vi "SavedSignal.vi"(11 "File selected":T2) -> (1 "Settings out":T1={"Name of test"="", "Date"=timestamp(0 s since 1904-01-01), "Location"="", "Template"="", "Soundcard"="", "resolution"=32, "Sampling rate"=48000, "Ch1 Gain "=0.0, "Ch2 Gain"=0.0, "Sample time (s)"=0.3, "Pre-trigger (s)"=0.01, "Hammer Threshold"=0.01, "Positions"=12, "Taps/Position"=5, "Set Names"="", "Freq resolution"=1.0, "Hammer cutoff"=1.0, "Mic cutoff"=1.0, "Double bounce "=0.0, "Hammer Cal"=1.0, "dB Offset"=0.0, "Accel Cal"=10.0, "Vibrometer Cal"=0.0, "Mic Cal"=1.0, "Output"=2, "Voltage Cal"=1.0, "Vibrometer Port"="ASRL27::INSTR", "Range"=10, "High Pass"=2, "Bandwidth"=25, "X Range"=[], "Y Range"=[], "dB Spread"=40.0, "Trigger"=0, "Ch_1"=1, "Ch_2"=2, "flip?"=FALSE, "60Hz"=FALSE, "Time offset"=0.0, "Piezo Cal"=1.0, "Default Notes"=""} {"Ch_2" min=1 step=1; "Ch_1" min=1 max=100 step=1; "Trigger" items=["Hammer (force)", "Self-tap", "Spacebar"]; "Bandwidth" items=["1 kHz"=1, "5 kHz"=5, "10 kHz"=10, "25 kHz"=25, "50 kHz"=50, "100 kHz"=100]; "High Pass" items=["Off", "13 Hz", "104 Hz"]; "Range" items=["10 mm/s"=1, "20 mm/s"=2, "50 mm/s"=5, "100 mm/s"=10, "200 mm/s"=20, "500 mm/s"=50, "1 m/s"=100, "2 m/s"=200]; "Output" items=["Accelerometer", "Speed (from acceleration)", "Microphone", "Vibrometer", "Piezo"]; "Voltage Cal" format="%#_13g"; "Ch2 Gain" format="%#_13g"; "Ch1 Gain" format="%#_13g"; "Double bounce" min=0.0; "Mic cutoff" min=0.0 format="%#_4g"; "Hammer cutoff" min=0.0 format="%#_4g"; "Freq resolution" min=0.0; "Pre-trigger (s)" format="%#_13g"; "Date" format="%<%H:%M\n%d/%m/%y>T"; "resolution" items=["16 bit"=16, "24 bit"=24, "32 bit"=32]; "Sampling rate" items=["22050 samp/s"=22050, "44100 samp/s"=44100, "48000 samp/s"=48000]}, 3 "update?":bool)   [LabVIEW 2022 SP3]
uses:
  ViolinSubs/PreferencesControl.ctl
  ViolinSubs/Curtin1_Label.ctl
  ViolinSubs/Mic/Mic_Global.vi
panel:
  out "Complex FRF":cluster{dbl, "df":dbl, cdb[]}
  out "starting settings":T1={"Name of test"="", "Date"=timestamp(0 s since 1904-01-01), "Location"="", "Template"="", "Soundcard"="", "resolution"=0, "Sampling rate"=0, "Ch1 Gain "=0.0, "Ch2 Gain"=0.0, "Sample time (s)"=0.0, "Pre-trigger (s)"=0.0, "Hammer Threshold"=0.0, "Positions"=0, "Taps/Position"=0, "Set Names"="", "Freq resolution"=0.0, "Hammer cutoff"=0.0, "Mic cutoff"=0.0, "Double bounce "=0.0, "Hammer Cal"=0.0, "dB Offset"=0.0, "Accel Cal"=0.0, "Vibrometer Cal"=0.0, "Mic Cal"=0.0, "Output"=0, "Voltage Cal"=0.0, "Vibrometer Port"="", "Range"=0, "High Pass"=0, "Bandwidth"=0, "X Range"=[], "Y Range"=[], "dB Spread"=0.0, "Trigger"=0, "Ch_1"=0, "Ch_2"=0, "flip?"=FALSE, "60Hz"=FALSE, "Time offset"=0.0, "Piezo Cal"=1.0, "Default Notes"=""} {"Ch_2" min=1 step=1; "Ch_1" min=1 max=100 step=1; "Trigger" items=["Hammer (force)", "Self-tap", "Spacebar"]; "Bandwidth" items=["1 kHz"=1, "5 kHz"=5, "10 kHz"=10, "25 kHz"=25, "50 kHz"=50, "100 kHz"=100]; "High Pass" items=["Off", "13 Hz", "104 Hz"]; "Range" items=["10 mm/s"=1, "20 mm/s"=2, "50 mm/s"=5, "100 mm/s"=10, "200 mm/s"=20, "500 mm/s"=50, "1 m/s"=100, "2 m/s"=200]; "Output" items=["Accelerometer", "Speed (from acceleration)", "Microphone", "Vibrometer", "Piezo"]; "Voltage Cal" format="%#_13g"; "Ch2 Gain" format="%#_13g"; "Ch1 Gain" format="%#_13g"; "Double bounce" min=0.0; "Mic cutoff" min=0.0 format="%#_4g"; "Hammer cutoff" min=0.0 format="%#_4g"; "Freq resolution" min=0.0; "Pre-trigger (s)" format="%#_13g"; "Date" format="%<%H:%M\n%d/%m/%y>T"; "resolution" items=["16 bit"=16, "24 bit"=24, "32 bit"=32]; "Sampling rate" items=["22050 samp/s"=22050, "44100 samp/s"=44100, "48000 samp/s"=48000]}
  out "path to settings file":path
  in  "Save as a Template":bool
  in  "Offset (msec)":dbl(slide) scale=0.0..10.0
  out "data":waveform(dbl)[](array[waveform])
  in  "Tab Control":enum32{"Raw", "Raw Calibrated", "Zoomed in"}(tab)
  out "Hammer":waveform(dbl)[](graph)
  out "Microphone":waveform(dbl)[](graph)
  out "Cal Hammer":waveform(dbl)[](graph)
  out "cal Mic":waveform(dbl)[](graph)
  out "Trig Mic":waveform(dbl)[](graph)
  out "Trig Hammer":waveform(dbl)[](graph)
  out "Average FRF":cluster{dbl, "df":dbl, dbl[]}(graph)
  out "Real/Imag":cluster{dbl, "df":dbl, dbl[]}[](graph)
  in  "Settings":T1={"Name of test"="", "Date"=timestamp(0 s since 1904-01-01), "Location"="", "Template"="", "Soundcard"="", "resolution"=32, "Sampling rate"=48000, "Ch1 Gain "=0.0, "Ch2 Gain"=0.0, "Sample time (s)"=0.3, "Pre-trigger (s)"=0.01, "Hammer Threshold"=0.01, "Positions"=12, "Taps/Position"=5, "Set Names"="", "Freq resolution"=1.0, "Hammer cutoff"=1.0, "Mic cutoff"=1.0, "Double bounce "=0.0, "Hammer Cal"=1.0, "dB Offset"=0.0, "Accel Cal"=10.0, "Vibrometer Cal"=0.0, "Mic Cal"=1.0, "Output"=2, "Voltage Cal"=1.0, "Vibrometer Port"="ASRL27::INSTR", "Range"=10, "High Pass"=2, "Bandwidth"=25, "X Range"=[], "Y Range"=[], "dB Spread"=40.0, "Trigger"=0, "Ch_1"=1, "Ch_2"=2, "flip?"=FALSE, "60Hz"=FALSE, "Time offset"=0.0, "Piezo Cal"=1.0, "Default Notes"=""} {"Ch_2" min=1 step=1; "Ch_1" min=1 max=100 step=1; "Trigger" items=["Hammer (force)", "Self-tap", "Spacebar"]; "Bandwidth" items=["1 kHz"=1, "5 kHz"=5, "10 kHz"=10, "25 kHz"=25, "50 kHz"=50, "100 kHz"=100]; "High Pass" items=["Off", "13 Hz", "104 Hz"]; "Range" items=["10 mm/s"=1, "20 mm/s"=2, "50 mm/s"=5, "100 mm/s"=10, "200 mm/s"=20, "500 mm/s"=50, "1 m/s"=100, "2 m/s"=200]; "Output" items=["Accelerometer", "Speed (from acceleration)", "Microphone", "Vibrometer", "Piezo"]; "Voltage Cal" format="%#_13g"; "Ch2 Gain" format="%#_13g"; "Ch1 Gain" format="%#_13g"; "Double bounce" min=0.0; "Mic cutoff" min=0.0 format="%#_4g"; "Hammer cutoff" min=0.0 format="%#_4g"; "Freq resolution" min=0.0; "Pre-trigger (s)" format="%#_13g"; "Date" format="%<%H:%M\n%d/%m/%y>T"; "resolution" items=["16 bit"=16, "24 bit"=24, "32 bit"=32]; "Sampling rate" items=["22050 samp/s"=22050, "44100 samp/s"=44100, "48000 samp/s"=48000]}
  # "Hz"
  # "dB"
  # "dB"
  # "sec"
  # "sec"
  # "mV/Pa"
  # "mV/m/s2"
  # "mV/mm/s"
  # "V/N"
  # "sec"
  # "sec"
  # "mV/N"
  # "a.u."
  # "a.u."
  # "sec"
  # "Hz"
  # "dB"
  # "dB"
  # "sec"
  # "sec"
  # "mV/Pa"
  # "mV/m/s2"
  # "mV/mm/s"
  # "V/N"
  # "sec"
  # "sec"
  # "mV/N"
  # "a.u."
  # "a.u."
  # "sec"
  # "Raw values from the Soundcard"
  # "Calibrated Values"
  # "Hz"
  # "dB"
  # "dB"
  # "sec"
  # "sec"
  # "mV/Pa"
  # "mV/m/s2"
  # "mV/mm/s"
  # "V/N"
  # "sec"
  # "sec"
  # "mV/N"
  # "a.u."
  # "a.u."
  # "sec"
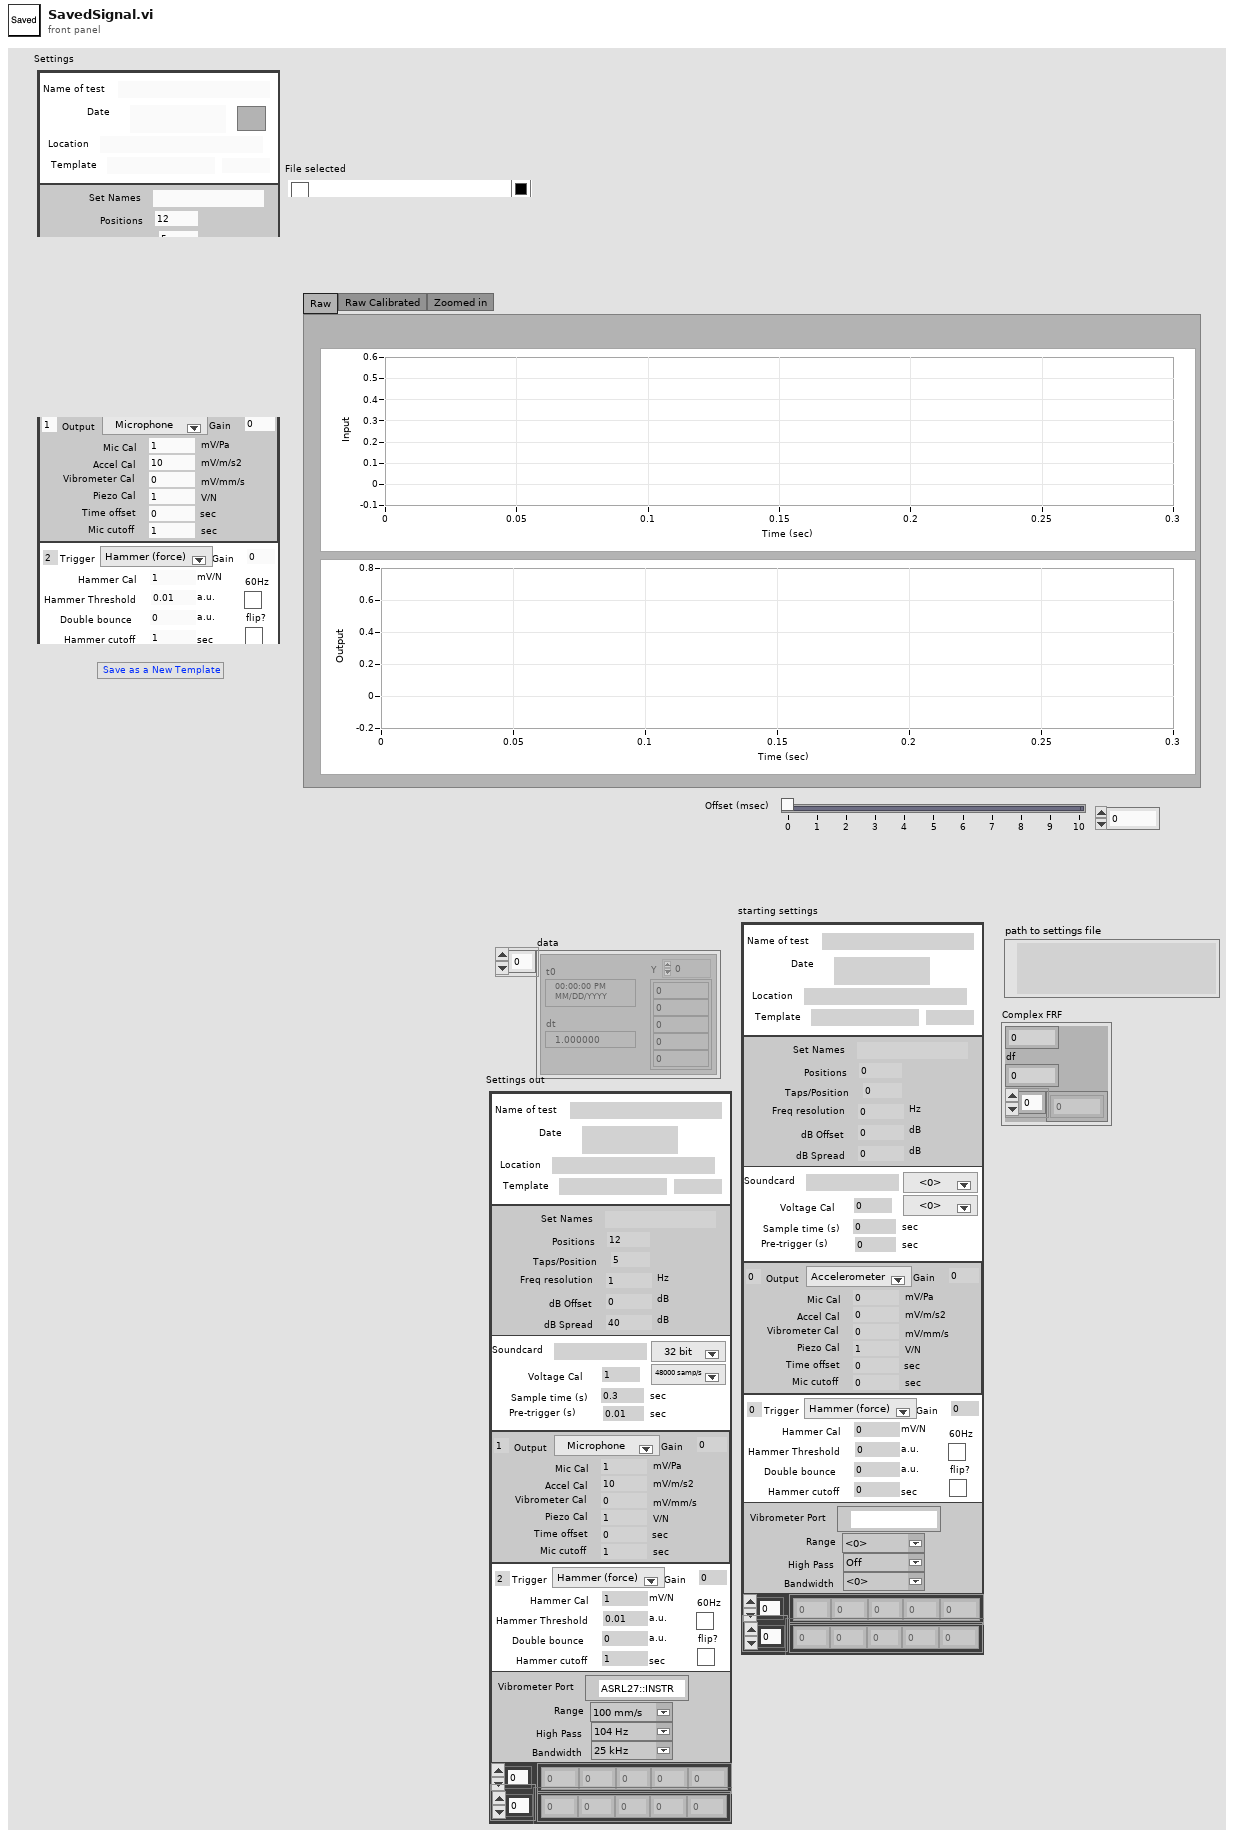
[diagram p1: front panel]
types:
  T1 = typedef "PreferencesControl.ctl" = cluster{"Name of test":string, "Date":timestamp, "Location":string, "Template":string, "Soundcard":string, "resolution":u16, "Sampling rate":u16, "Ch1 Gain ":dbl, "Ch2 Gain":dbl, "Sample time (s)":dbl, "Pre-trigger (s)":dbl, "Hammer Threshold":dbl, "Positions":i16, "Taps/Position":i16, "Set Names":string, "Freq resolution":dbl, "Hammer cutoff":dbl, "Mic cutoff":dbl, "Double bounce ":dbl, "Hammer Cal":dbl, "dB Offset":dbl, "Accel Cal":dbl, "Vibrometer Cal":dbl, "Mic Cal":dbl, "Output":u16, "Voltage Cal":dbl, "Vibrometer Port":refnum<visa-resource-name>, "Range":u16, "High Pass":u16, "Bandwidth":u16, "X Range":cluster{"Minimum":dbl, "Maximum":dbl, "Increment":dbl, "Minor Increment":dbl, "Start":dbl}[], "Y Range":cluster{"Minimum":dbl, "Maximum":dbl, "Increment":dbl, "Minor Increment":dbl, "Start":dbl}[], "dB Spread":dbl, "Trigger":u16, "Ch_1":u8, "Ch_2":u8, "flip?":bool, "60Hz":bool, "Time offset":dbl, "Piezo Cal":dbl, "Default Notes":string}
  T2 = typedef "Curtin1_Label.ctl" = cluster{"Show?":bool, "Name":string, "Color":u32, "Path":path, "Show Notes":bool}
  T3 = enum32{"Invalid", "Default", "Floating", "Floating/Auto-Hide", "Modal"}
  T4 = enum8{"Enabled", "Disabled", "Disabled and Grayed Out"}
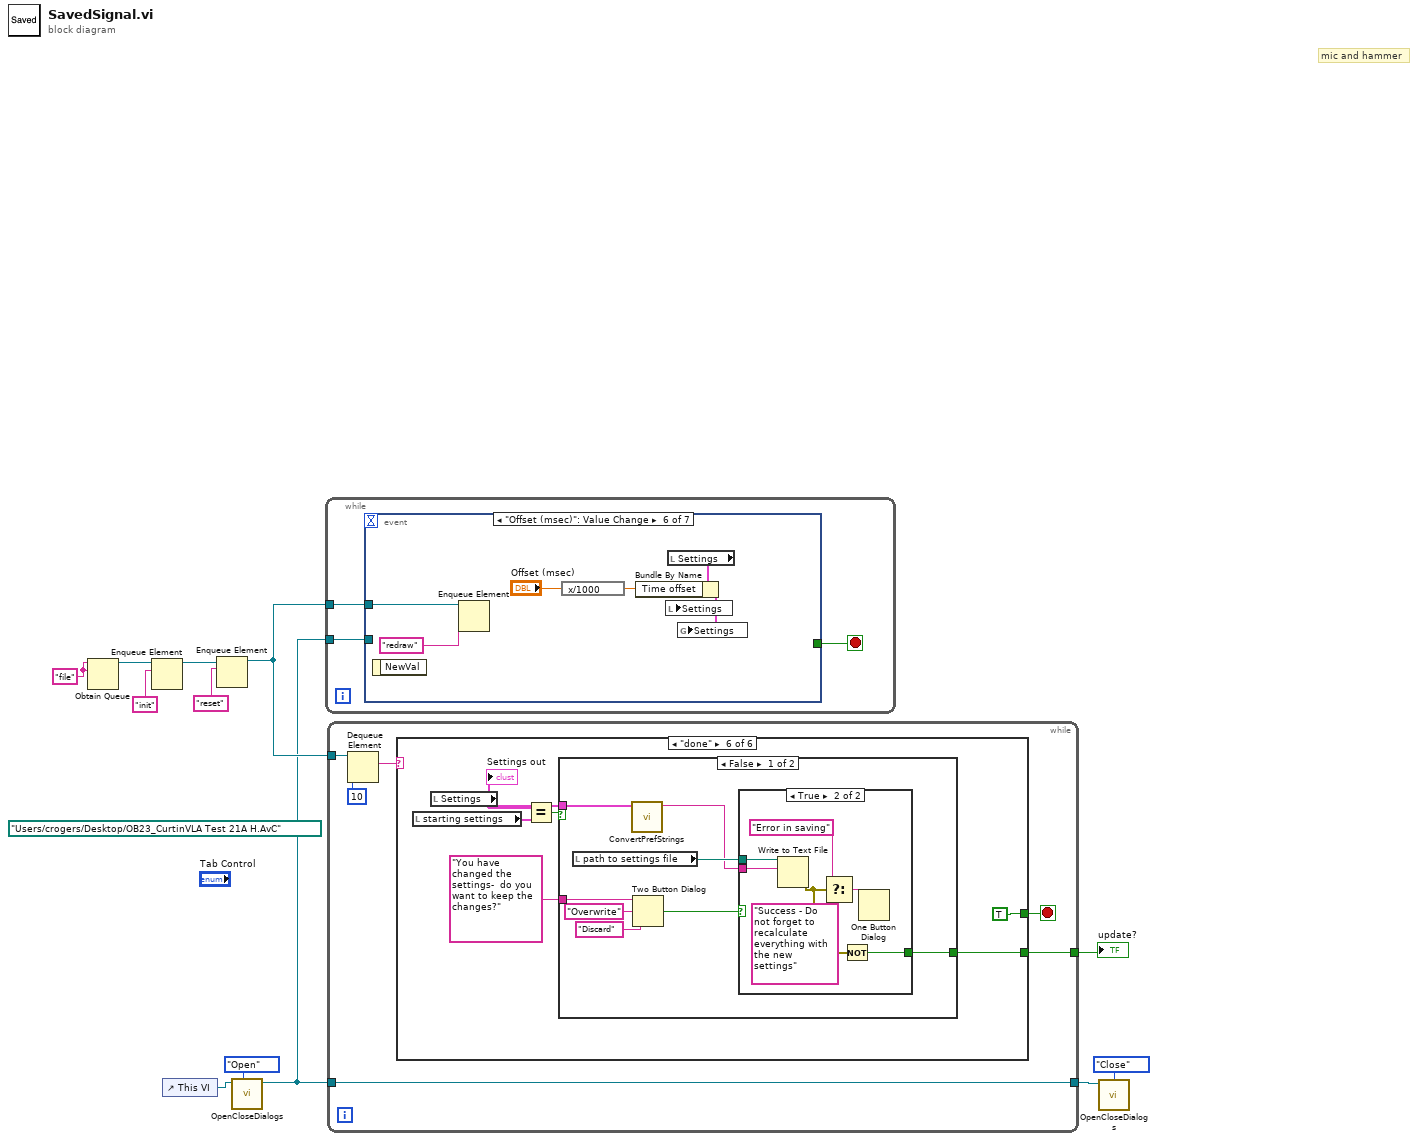
[diagram p0: block diagram]
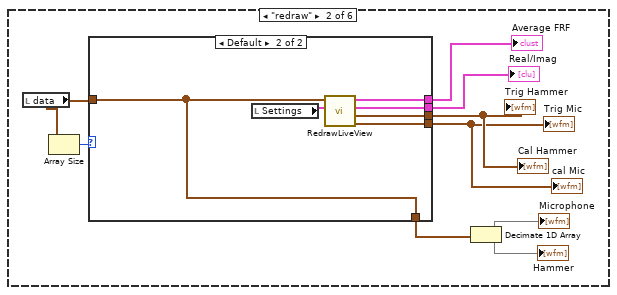
[diagram p3: hidden frame]
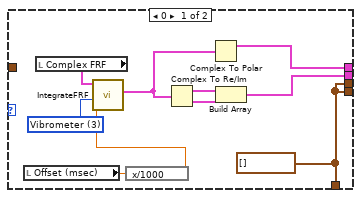
[diagram p4: hidden frame]
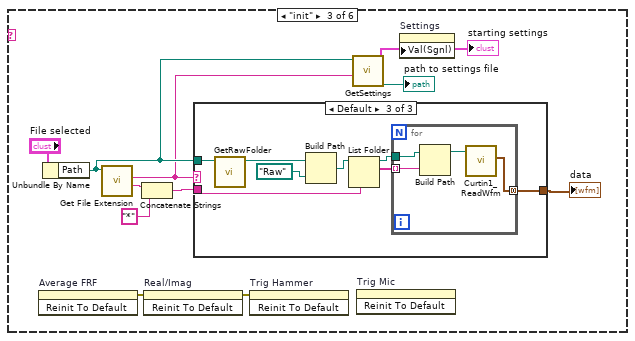
[diagram p5: hidden frame]
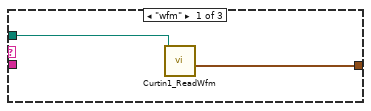
[diagram p6: hidden frame]
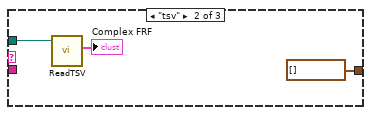
[diagram p7: hidden frame]
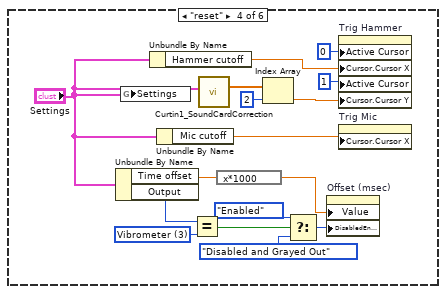
[diagram p8: hidden frame]
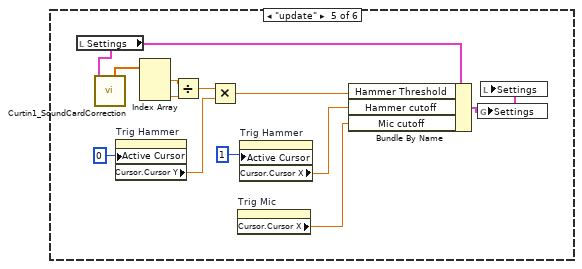
[diagram p9: hidden frame]
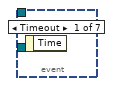
[diagram p12: hidden frame]
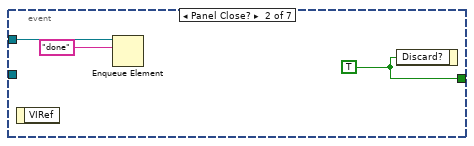
[diagram p13: hidden frame]
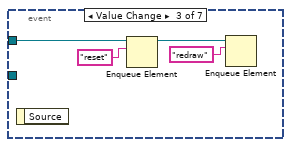
[diagram p14: hidden frame]
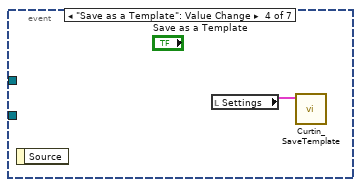
[diagram p15: hidden frame]
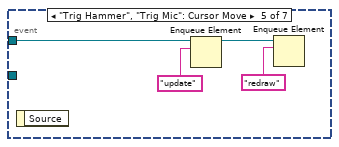
[diagram p16: hidden frame]
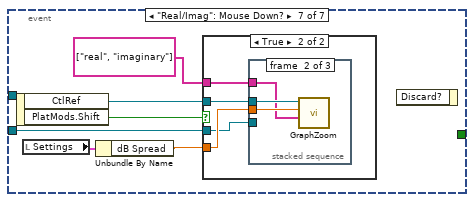
[diagram p17: hidden frame]
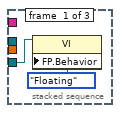
[diagram p19: hidden frame]
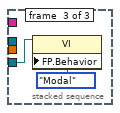
[diagram p20: hidden frame]
diagram:
  (unwired) path "/Users/crogers/Desktop/OB23_CurtinVLA Test 21A H.AvC" ("Path")
  w6 = "file" ("name (unnamed)")
  # "mic and hammer"
  n1 = Obtain Queue(name (unnamed)=w6, element data type=w6) -> (queue out=w5:refnum<queue>)  [unwired: 3 in, 2 out]
  n2 = Enqueue Element(queue=w5, element="init") -> (queue out=w8:refnum<queue>)  [unwired: 2 in, 2 out]
  n3 = control-ref of="This VI"() -> (w3:refnum<vi>)
  n4 = Enqueue Element(queue=w8, element="reset") -> (queue out=w7:refnum<queue>)  [unwired: 2 in, 2 out]
  n5 = call "OpenCloseDialogs.vi"("Task"=enum16{"Open", "Close"}."Open", "VI in"=w3) -> ("VI out"=w2:refnum<vi>)  [unwired: 8 in, 1 out]
  n6 = while {
    tunnel: w7 -> [w15]
    tunnel: w2 -> [w13]
    stop <- w14 stop-if-true
    n7 = event shown="[5] \"Offset (msec)\": Value Change" {
      selector: _ -> [_ _ _ _ _ _ _]
      dyn-events: _ -> [_ _ _ _ _ _ _]
      timeout: _ -> [_ _ _ _ _ _ _]
      tunnel: [_ w18 _ _ _ _ _] -> w14
      tunnel: w15 -> [_ w17 w22 _ w26 w28 _]
      tunnel: w13 -> [_ _ _ _ _ _ w35]
      event Timeout {
        n8 = event-data() -> ()  [unwired: 1 in, 1 out]
      }
      event Panel Close? {
        w18 = TRUE ("Discard?")
        n9 = event-data() -> ()  [unwired: 1 in, 1 out]
        n10 = Enqueue Element(queue=w17, element="done") -> ()  [unwired: 2 in, 3 out]
        n11 = event-data("Discard?"=w18) -> ()  [unwired: 1 in, 1 out]
      }
      event Value Change {
        n12 = event-data() -> ()  [unwired: 1 in, 1 out]
        n13 = Enqueue Element(queue=w22, element="reset") -> (queue out=w20:refnum<queue>)  [unwired: 2 in, 2 out]
        n14 = Enqueue Element(queue=w20, element="redraw") -> ()  [unwired: 2 in, 3 out]
      }
      event "Save as a Template": Value Change {
        n15 = event-data() -> ()  [unwired: 1 in, 1 out]
        n16 = local read "Settings"() -> (w23:T1)
        n17 = call "Curtin_SaveTemplate.vi"("Settings in"=w23) -> ()  [unwired: 8 in, 3 out]
      }
      event "Trig Hammer", "Trig Mic": Cursor Move {
        n18 = event-data() -> ()  [unwired: 1 in, 1 out]
        n19 = Enqueue Element(queue=w26, element="update") -> (queue out=w24:refnum<queue>)  [unwired: 2 in, 2 out]
        n20 = Enqueue Element(queue=w24, element="redraw") -> ()  [unwired: 2 in, 3 out]
      }
      event "Offset (msec)": Value Change {
        n21 = event-data() -> ()  [unwired: 1 in, 1 out]
        n22 = Enqueue Element(queue=w28, element="redraw") -> ()  [unwired: 2 in, 3 out]
        n23 = expression code="x/1000"("Offset (msec)") -> (w30:dbl)
        n24 = local read "Settings"() -> (w33:T1)
        n25 = Bundle By Name(cluster=w33, "Time offset"=w30) -> (w32:T1)
        n26 = local write "Settings"(w32) -> ()
        n27 = global write "Mic_Global.vi" "Settings"(w32) -> ()
      }
      event "Real/Imag": Mouse Down? {
        n28 = event-data() -> ("CtlRef"=w38:refnum<vi>, "PlatMods.Shift"=w39:bool)  [unwired: 1 in]
        n29 = local read "Settings"() -> (w37:T1)
        n30 = Unbundle By Name(w37) -> ("dB Spread"=w36:dbl)
        n31 = case shown="True" w39 {
          tunnel: w38 -> [_ w43]
          tunnel: w36 -> [_ w42]
          tunnel: w35 -> [_ w41]
          tunnel: string[] ["real", "imaginary"] -> [_ w40]
          frame False {
          }
          frame True {
            n32 = stacked-sequence {
              tunnel: w43 -> [_ w48 _]
              tunnel: w42 -> [_ w47 _]
              tunnel: w41 -> [w44 _ w49]
              tunnel: w40 -> [_ w46 _]
              frame #0 {
                n33 = property class="VI"(reference=w44, "FP.Behavior"=T3."Floating" ("Front Panel Window:Behavior")) -> ()  [unwired: 1 in, 2 out]
              }
              frame #1 {
                n34 = call "GraphZoom.vi"("Names"=w46, "dB Range"=w47, "Graph"=w48) -> ()  [unwired: 9 in]
              }
              frame #2 {
                n35 = property class="VI"(reference=w49, "FP.Behavior"=T3."Modal" ("Front Panel Window:Behavior")) -> ()  [unwired: 1 in, 2 out]
              }
            }
          }
        }
        n36 = event-data() -> ()  [unwired: 2 in, 1 out]
      }
    }
  }
  n37 = while {
    tunnel: w7 -> [w56]
    tunnel: [w52] -> w10
    tunnel: w2 -> [w52]
    tunnel: [w51] -> w1
    stop <- w53 stop-if-true
    n38 = Dequeue Element(queue=w56, timeout in ms (-1)=10) -> (element=w55:string)  [unwired: 1 in, 3 out]
    n39 = case shown="\"done\"" w55 {
      tunnel: [_ _ _ _ _ TRUE ("Discard?")] -> w53
      tunnel: [_ _ _ _ _ w138] -> w51
      frame Default {
      }
      frame "redraw" {
        n40 = local read "data"() -> (w58:waveform(dbl)[])
        n41 = Array Size(array=w58) -> (size(s)=w57:i32)
        n42 = case shown="Default" w57 {
          tunnel: [w66 w80] -> w65
          tunnel: [w74 w79] -> w64
          tunnel: w58 -> [_ w76]
          tunnel: [w75 w78] -> w63
          tunnel: [w75 w77] -> w62
          tunnel: [w75 w76] -> w59
          frame 0 {
            w71 = u16 3 items=["Accelerometer", "Accel (speed)", "Microphone", "Vibrometer"] ("Output")
            w75 = waveform(dbl)[] [] ("Trig Hammer")
            n43 = local read "Offset (msec)"() -> (w72:dbl)
            n44 = local read "Complex FRF"() -> (w70:cluster{dbl, "df":dbl, cdb[]})
            n45 = expression code="x/1000"(w72) -> (w73:dbl)
            n46 = call "IntegrateFRF.vi"("delay (sec)"=w73, "Output"=w71, "Complex FRF"=w70) -> ("Complex FRF out"=w69:cluster{"t0":dbl, "dt":dbl, "Y":cdb[]})  [unwired: 7 in, 1 out]
            n47 = Complex To Re/Im(x + iy=w69) -> (x=w68:cluster{"t0":dbl, "dt":dbl, "Y":dbl[]}, y=w67:cluster{"t0":dbl, "dt":dbl, "Y":dbl[]})
            n48 = Complex To Polar(r * e^(i*theta)=w69) -> (r=w66:cluster{"t0":dbl, "dt":dbl, "Y":dbl[]})  [unwired: 1 out]
            n49 = Build Array(w68, w67) -> (w74:cluster{"t0":dbl, "dt":dbl, "Y":dbl[]}[])
          }
          frame Default {
            n50 = local read "Settings"() -> (w81:T1)
            n51 = call "RedrawLiveView.vi"("Settings"=w81, "data"=w76) -> ("Trig Mic"=w77:waveform(dbl)[], "Trig Hammer"=w78:waveform(dbl)[], "Real/Imag"=w79:cluster{dbl, "df":dbl, dbl[]}[], "Average FRF"=w80:cluster{dbl, "df":dbl, dbl[]})  [unwired: 6 in]
          }
        }
        "Trig Hammer" <- w63
        "Trig Mic" <- w62
        "Real/Imag" <- w64
        "Average FRF" <- w65
        "Cal Hammer" <- w63
        "cal Mic" <- w62
        n52 = Decimate 1D Array(w59) -> (→"Microphone":waveform(dbl)[], →"Hammer":waveform(dbl)[])
      }
      frame "init" {
        n53 = invoke on="Average FRF" class="WFGraph (strict)" method="Reinit To Default"() -> (error out=w84:errorcluster)  [unwired: 3 in, 2 out]
        n54 = Unbundle By Name("File selected") -> ("Path"=w89:path)
        n55 = call <vilib>:"Get File Extension.vi"("file"=w89) -> ("filename without extension"=w91:string, "lowercase file extension"=w88:string)  [unwired: 6 in, 3 out]
        n56 = Concatenate Strings(w91, "*" ("string")) -> (w92:string)
        n57 = invoke on="Real/Imag" class="WFGraph (strict)" method="Reinit To Default"(error in=w84) -> (error out=w85:errorcluster)  [unwired: 2 in, 2 out]
        n58 = case shown="Default" w88 {
          tunnel: w89 -> [w94 w97 w105]
          tunnel: w92 -> [_ _ w104]
          tunnel: [w93 waveform(dbl)[] [] ("all waveforms in record") w98] -> w82
          frame "wfm" {
            n59 = call "Curtin1_ReadWfm.vi"("appended path"=w94) -> ("all waveforms in record"=w93:waveform(dbl)[])  [unwired: 9 in, 1 out]
          }
          frame "tsv" {
            n60 = call "ReadTSV.vi"("Path"=w97) -> ("Complex FRF"=→"Complex FRF":cluster{dbl, "df":dbl, cdb[]})  [unwired: 9 in, 1 out]
          }
          frame Default {
            n61 = call "GetRawFolder.vi"("File name"=w105) -> ("Path to Raw data"=w100:path)  [unwired: 10 in]
            n62 = Build Path(base path=w100, name or relative path=path "Raw") -> (appended path=w99:path)
            n63 = List Folder(path=w99, pattern=w104) -> (path out=w103:path, filenames=w102:string[])  [unwired: 2 in, 2 out]
            n64 = for {
              tunnel: w103 -> [w109]
              tunnel: w102 -> [w108] mode=indexing
              tunnel: [w107] -> w98 mode=concatenating
              n65 = Build Path(base path=w109, name or relative path=w108) -> (appended path=w106:path)
              n66 = call "Curtin1_ReadWfm.vi"("appended path"=w106) -> ("all waveforms in record"=w107:waveform(dbl)[])  [unwired: 9 in, 1 out]
            }
          }
        }
        "data" <- w82
        n67 = invoke on="Trig Hammer" class="WFGraph (strict)" method="Reinit To Default"(error in=w85) -> ()  [unwired: 2 in, 3 out]
        n68 = call "GetSettings.vi"("lowercase file extension"=w88, "wavform file"=w89) -> ("path to settings file"=→"path to settings file":path, "Settings"=w90:T1)  [unwired: 8 in]
        "starting settings" <- w90
        n69 = invoke on="Trig Mic" class="WFGraph (strict)" method="Reinit To Default"() -> ()  [unwired: 3 in, 3 out]
        n70 = property on="Settings" class="Clust (strict)"("Val(Sgnl)"=w90) -> ()  [unwired: 2 in, 2 out]
      }
      frame "reset" {
        w117 = u16 3 items=["Accelerometer", "Accel (speed)", "Microphone", "Vibrometer"] ("Output")
        n71 = Unbundle By Name("Settings") -> ("Time offset"=w120:dbl, "Output"=w125:u16)
        n72 = global write "Mic_Global.vi" "Settings"("Settings") -> ()
        n73 = Unbundle By Name("Settings") -> ("Hammer cutoff"=w113:dbl)
        n74 = Unbundle By Name("Settings") -> ("Mic cutoff"=w110:dbl)
        n75 = Equal?(x=w125, y=w117) -> (x = y?=w124:bool)
        n76 = call "Curtin1_SoundCardCorrection.vi"("Settings"="Settings") -> ("Converted"=w121:dbl[])  [unwired: 5 in, 5 out]
        n77 = expression code="x*1000"(w120) -> (w112:dbl)
        n78 = Index Array(array=w121, index=2) -> (element=w122:dbl)
        n79 = Select(t=T4."Enabled" ("Disabled"), s=w124, f=T4."Disabled and Grayed Out" ("Disabled")) -> (s? t:f=w123:T4)
        n80 = property on="Offset (msec)" class="Slide (strict)"("Value"=w112, "DisabledEnum"=w123) -> ()  [unwired: 2 in, 2 out]
        n81 = property on="Trig Hammer" class="WFGraph (strict)"("Active Cursor"=u32 0, "Cursor.Cursor X"=w113, "Active Cursor"=u32 1, "Cursor.Cursor Y"=w122) -> ()  [unwired: 2 in, 2 out]
        n82 = property on="Trig Mic" class="WFGraph (strict)"("Cursor.Cursor X"=w110) -> ()  [unwired: 2 in, 2 out]
      }
      frame "update" {
        n83 = local read "Settings"() -> (w136:T1)
        n84 = call "Curtin1_SoundCardCorrection.vi"("Settings"=w136) -> ("Converted"=w130:dbl[])  [unwired: 5 in, 5 out]
        n85 = property on="Trig Hammer" class="WFGraph (strict)"("Active Cursor"=u32 0) -> ("Cursor.Cursor Y"=w134:dbl)  [unwired: 2 in, 2 out]
        n86 = Index Array(array=w130) -> (element #1=w131:dbl, element #3=w132:dbl)  [unwired: 3 in, 1 out]
        n87 = Divide(x=w131, y=w132) -> (x/y=w133:dbl)
        n88 = Multiply(x=w133, y=w134) -> (x*y=w135:dbl)
        n89 = property on="Trig Mic" class="WFGraph (strict)"() -> ("Cursor.Cursor X"=w126:dbl)  [unwired: 2 in, 2 out]
        n90 = property on="Trig Hammer" class="WFGraph (strict)"("Active Cursor"=u32 1) -> ("Cursor.Cursor X"=w137:dbl)  [unwired: 2 in, 2 out]
        n91 = Bundle By Name(cluster=w136, "Hammer Threshold"=w135, "Hammer cutoff"=w137, "Mic cutoff"=w126) -> (w129:T1)
        n92 = global write "Mic_Global.vi" "Settings"(w129) -> ()
        n93 = local write "Settings"(w129) -> ()
      }
      frame "done" {
        n94 = local read "starting settings"() -> (w142:T1)
        n95 = local read "Settings"() -> (w139:T1)
        "Settings out" <- w139
        n96 = Equal?(x=w139, y=w142) -> (x = y?=w141:bool)
        n97 = case shown="False" w141 {
          tunnel: "You have changed the settings-  do you want to keep the changes?" ("message") -> [w151 _]
          tunnel: w139 -> [w148 _]
          tunnel: [w144 _] -> w138
          frame False {
            n98 = local read "path to settings file"() -> (w147:path)
            n99 = call "ConvertPrefStrings.vi"("Settings"=w148) -> ("String Out"=w146:string)  [unwired: 9 in, 1 out]
            n100 = Two Button Dialog(message=w151, 1:"Discard" ("F button name (\"Cancel\")"), 2:"Overwrite" ("T button name (\"OK\")")) -> (T button?=w145:bool)
            n101 = case shown="True" w145 {
              tunnel: w147 -> [_ w158]
              tunnel: w146 -> [_ w157]
              tunnel: [_ w152] -> w144
              frame False {
              }
              frame True {
                n102 = Write to Text File(file (use dialog)=w158, text=w157) -> (error out=w153:errorcluster)  [unwired: 2 in, 2 out]
                n103 = Select(t="Error in saving" ("F button name (\"Cancel\")"), s=w153, f="Success - Do not forget to recalculate everything with the new settings" ("F button name (\"Cancel\")")) -> (s? t:f=w155:string)
                n104 = Not(x=w153) -> (.not. x?=w152:bool)
                n105 = One Button Dialog(message=w155) -> ()  [unwired: 1 in, 1 out]
              }
            }
          }
          frame True {
          }
        }
      }
    }
  }
  "update?" <- w1
  n106 = call "OpenCloseDialogs.vi"("Task"=enum16{"Open", "Close"}."Close", "VI in"=w10) -> ()  [unwired: 8 in, 2 out]
